vi "PC_CallTestRT.vi"() -> ()   [LabVIEW 2010]
panel:
  out "Control Value:Get All":cluster{"Name":string, "Variant Data":variant}[](array[cluster])
  out "error out 2":errorcluster
  out "error out":errorcluster
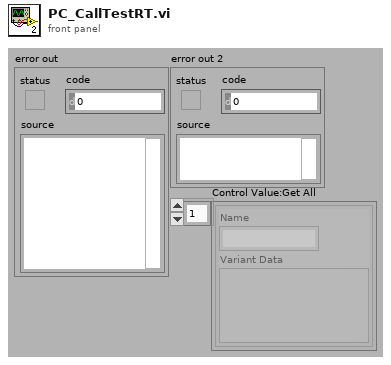
[diagram p1: front panel]
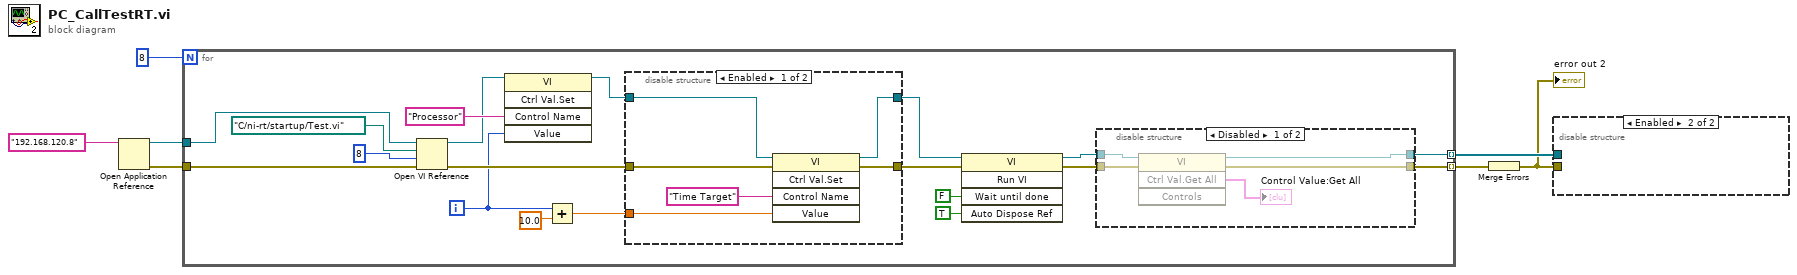
[diagram p0: block diagram]
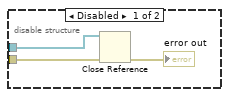
[diagram p2: hidden frame]
diagram:
  n1 = Open Application Reference(11:"192.168.120.8" ("machine name (\"\":  open local reference)")) -> (0:w1:errorcluster, 3:w2:refnum<vi>)  [unwired: 3 in]
  n2 = for {
    N: 8 -> [_]
    tunnel: [w14] -> w7 mode=indexing
    tunnel: [w16] -> w6 mode=indexing
    tunnel: w2 -> [w20]
    tunnel: w1 -> [w19]
    i -> [w12]
    n3 = Open VI Reference(application reference (local)=w20, vi path=path "C:/ni-rt/startup/Test.vi", options=8, error in (no error)=w19) -> (vi reference=w11:refnum<vi>, error out=w25:errorcluster)  [unwired: 2 in]
    n4 = invoke class="VI" method="Ctrl Val.Set"(reference=w11, "Control Name"="Processor", "Value"=w12) -> (reference out=w10:refnum<vi>)  [unwired: 2 in, 4 out]
    n5 = Add(x=w12, y=10.0) -> (x+y=w9:dbl)
    n6 = disable-structure shown="Enabled" {
      disable-tunnel: w10 -> [w37 w39]
      disable-tunnel: w25 -> [w36 w38]
      disable-tunnel: [w35 w39] -> w24
      disable-tunnel: [w34 w38] -> w21
      disable-tunnel: w9 -> [w32 _]
      frame Enabled {
        n7 = invoke class="VI" method="Ctrl Val.Set"(reference=w37, error in=w36, "Control Name"="Time Target", "Value"=w32) -> (reference out=w35:refnum<vi>, error out=w34:errorcluster)  [unwired: 1 in, 3 out]
      }
      frame Disabled {
      }
    }
    n8 = invoke class="VI" method="Run VI"(reference=w24, error in=w21, "Wait until done"=FALSE ("Wait Until Done"), "Auto Dispose Ref"=TRUE ("Auto Dispose Reference")) -> (reference out=w17:refnum<vi>, error out=w15:errorcluster)  [unwired: 1 in, 3 out]
    n9 = disable-structure shown="Disabled" {
      disable-tunnel: w17 -> [w31 _]
      disable-tunnel: [w30 _] -> w16
      disable-tunnel: w15 -> [w29 _]
      disable-tunnel: [w28 _] -> w14
      frame Disabled {
        n10 = invoke class="VI" method="Ctrl Val.Get All"(reference=w31, error in=w29) -> (reference out=w30:refnum<vi>, error out=w28:errorcluster, "Get All Control Values Variant"=→"Control Value:Get All":cluster{"Name":string, "Variant Data":variant}[])  [unwired: 2 in, 1 out]
      }
      frame Enabled {
      }
    }
  }
  n11 = Merge Errors(w7) -> (w4:errorcluster)
  "error out 2" <- w4
  n12 = disable-structure shown="Enabled" {
    disable-tunnel: w6 -> [w42 _]
    disable-tunnel: w4 -> [w41 _]
    frame Disabled {
      n13 = Close Reference(reference=w42, error in (no error)=w41) -> (error out=→"error out":errorcluster)
    }
    frame Enabled {
    }
  }
